vi "display.vi"() -> ()   [LabVIEW 2010]
panel:
  out "x+1":i32
  out "data":string
  out "Waveform Graph":waveform(dbl)[](graph)
  in  "Array of Waveform":waveform(dbl)[](array[waveform])
  out "Event":string
  out "Variant":variant
  in  "Parameter":cluster{"Event":string, "Variant":variant}
  in  "Target IP Address":string="192.168.120.8"
  in  "Boolean":bool
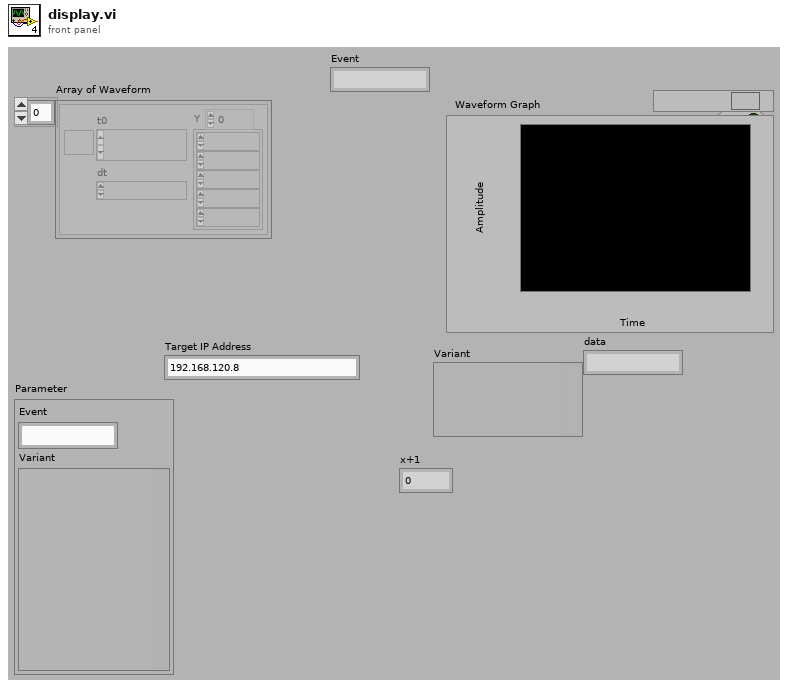
[diagram p1: front panel]
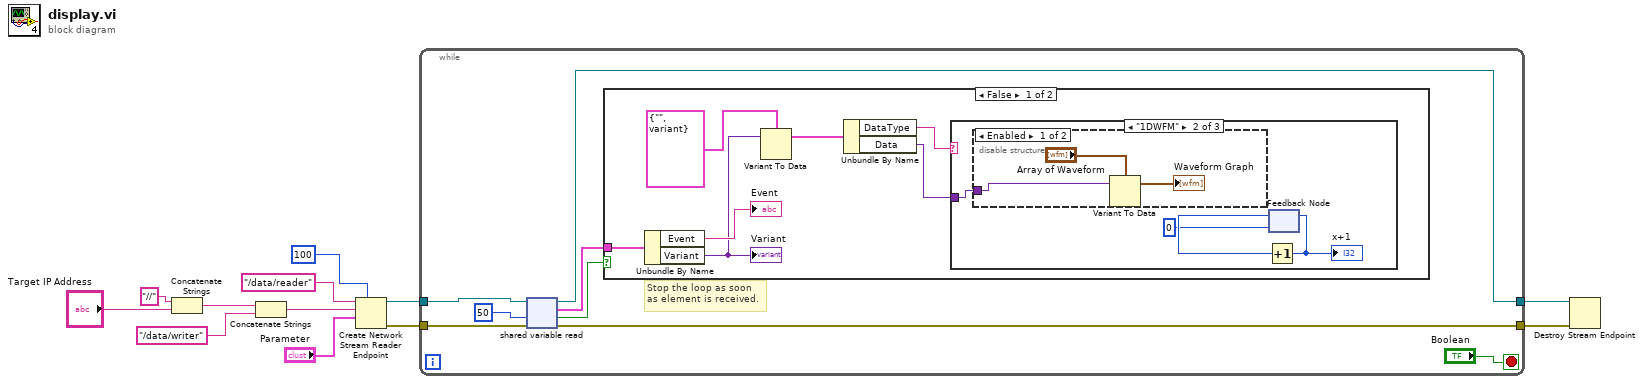
[diagram p0: block diagram]
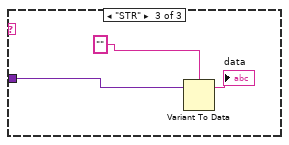
[diagram p4: hidden frame]
diagram:
  n1 = Concatenate Strings("//" ("reader url"), "Target IP Address") -> (w2:string)
  n2 = Concatenate Strings(w2, "/data/writer" ("reader url")) -> (w6:string)
  n3 = Create Network Stream Reader Endpoint(7:100 ("reader buffer size"), 9:"Parameter", 10:w6, 11:"/data/reader" ("writer name")) -> (0:w11:errorcluster, 3:w10:refnum<k21>)  [unwired: 2 in]
  n4 = while {
    tunnel: w11 -> [w20]
    tunnel: w10 -> [w19]
    tunnel: [w17] -> w9
    tunnel: [w16] -> w8
    stop <- "Boolean" stop-if-true
    # "Stop the loop as soon \nas element is received."
    n5 = shared-variable-read(w19, w20, 50 ("timeout ms")) -> (w16:refnum<k21>, w17:errorcluster, w13:bool, w15:cluster{"Event":string, "Variant":variant})
    n6 = case shown="False" w13 {
      tunnel: w15 -> [w27 _]
      frame False {
        n7 = Unbundle By Name(w27) -> ("Event"=→"Event":string, "Variant"=w24:variant)
        "Variant" <- w24
        n8 = Variant To Data(Variant=w24, type=cluster{"DataType":string, "Data":variant} {"DataType"="", "Data"=variant} ("cluster")) -> (data=w23:cluster{"DataType":string, "Data":variant})  [unwired: 1 in, 1 out]
        n9 = Unbundle By Name(w23) -> ("DataType"=w22:string, "Data"=w21:variant)
        n10 = case shown="\"1DWFM\"" w22 {
          tunnel: w21 -> [_ w31 w37]
          frame "False", Default {
          }
          frame "1DWFM" {
            n11 = disable-structure shown="Enabled" {
              disable-tunnel: w31 -> [w32 _]
              frame Enabled {
                n12 = Variant To Data(Variant=w32, type="Array of Waveform") -> (data=→"Waveform Graph":waveform(dbl)[])  [unwired: 1 in, 1 out]
              }
              frame Disabled {
              }
            }
            n13 = feedback #1(0) -> (w30:i32)
            n14 = Increment(x=w30) -> (x+1=w28:i32)
            "x+1" <- w28
            n15 = feedback-in #1(w28) -> ()
          }
          frame "STR" {
            n16 = Variant To Data(Variant=w37, type="") -> (data=→"data":string)  [unwired: 1 in, 1 out]
          }
        }
      }
      frame True {
      }
    }
  }
  n17 = Destroy Stream Endpoint(8:w9, 11:w8) -> ()  [unwired: 1 out]
